vi "extract orbit queue to time range.vi"(6 "most recent?":bool, 7 "recent interval":dbl=5.0, 8 "error in (no error)":errorcluster, 9 "t0":dbl=-1.0, 10 "t1":dbl=-1.0, 11 "orbit fit":refnum<queue>) -> (0 "error out":errorcluster, 2 "extracted elements":T1[](array[typedef]))   [LabVIEW 2017]
uses:
  typedefs/orbit parameters with crossing info.ctl
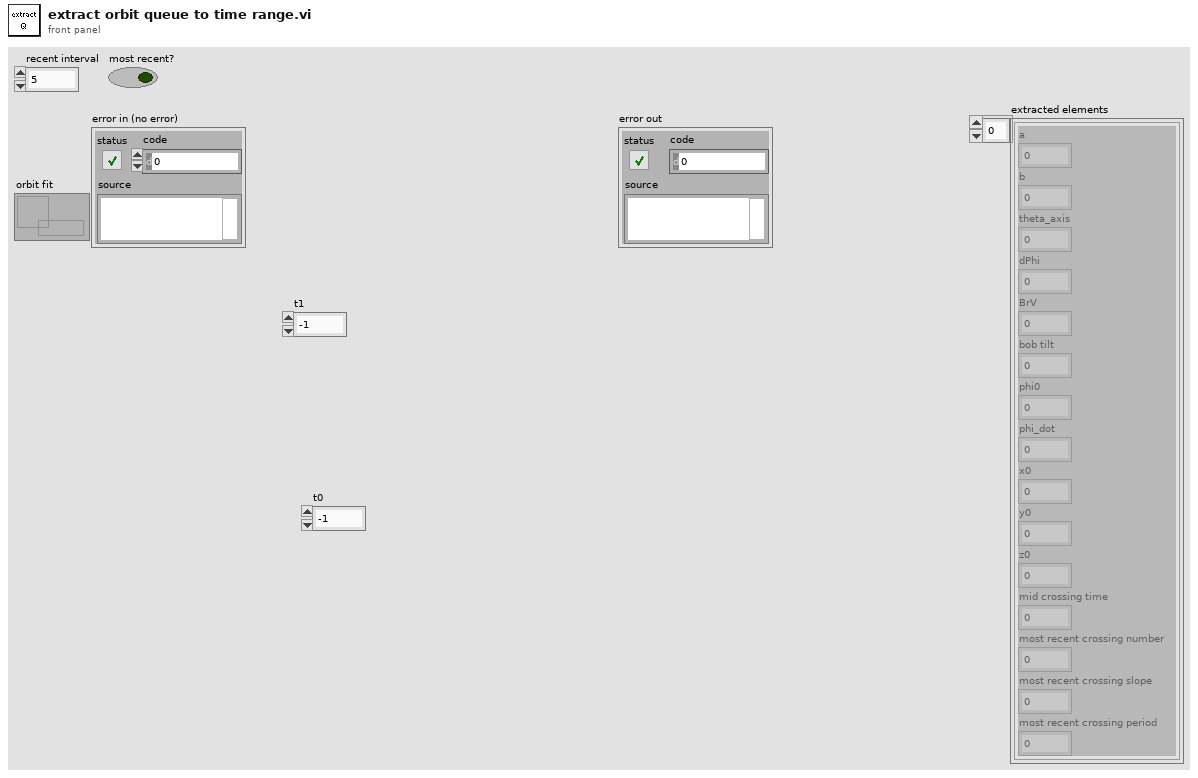
[diagram p1: front panel]
types:
  T1 = typedef "orbit parameters with crossing info.ctl" = cluster{"a":dbl, "b":dbl, "theta_axis":dbl, "dPhi":dbl, "BrV":dbl, "bob tilt":dbl, "phi0":dbl, "phi_dot":dbl, "x0":dbl, "y0":dbl, "z0":dbl, "mid crossing time":dbl, "most recent crossing number":dbl, "most recent crossing slope":dbl, "most recent crossing period":dbl}
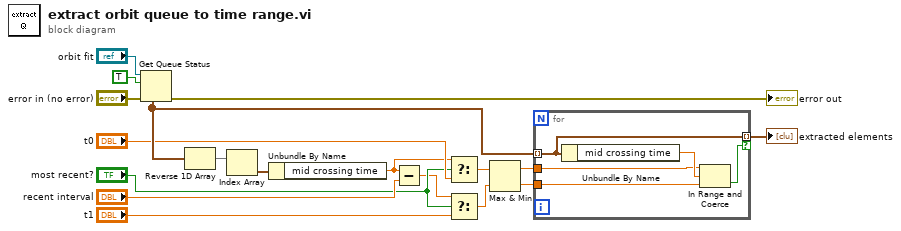
[diagram p0: block diagram]
diagram:
  n1 = Get Queue Status(queue="orbit fit", return elements? (F)=TRUE, error in (no error)="error in (no error)") -> (error out=→"error out":errorcluster, elements=w14:T1[])  [unwired: 6 out]
  n2 = Reverse 1D Array(array=w14) -> (reversed array=w13:T1[])
  n3 = Index Array(array=w13) -> (element=w12:T1)  [unwired: 1 in]
  n4 = Unbundle By Name(w12) -> ("mid crossing time"=w10:dbl)
  n5 = Subtract(x=w10, y="recent interval") -> (x-y=w7:dbl)
  n6 = Select(t=w10, s="most recent?", f="t0") -> (s? t:f=w5:dbl)
  n7 = Select(t=w7, s="most recent?", f="t1") -> (s? t:f=w4:dbl)
  n8 = Max & Min(x=w5, y=w4) -> (max(x,y)=w3:dbl, min(x,y)=w2:dbl)
  n9 = for {
    tunnel: w14 -> [w23] mode=indexing
    tunnel: [w23] -> w1 mode=indexing if=w21
    tunnel: w3 -> [w20]
    tunnel: w2 -> [w19]
    n10 = Unbundle By Name(w23) -> ("mid crossing time"=w22:dbl)
    n11 = In Range and Coerce(upper limit=w20, x=w22, lower limit=w19) -> (In Range?=w21:bool)  [unwired: 1 out]
  }
  "extracted elements" <- w1
